vi "enqueue states.vi"(8 "error in (no error)":errorcluster, 10 "Wash Options":T1, 11 "Queue in":refnum<queue>) -> (0 "error out":errorcluster)   [LabVIEW 2015]
uses:
  Controls/Wash Options.ctl
  Controls/#status.ctl
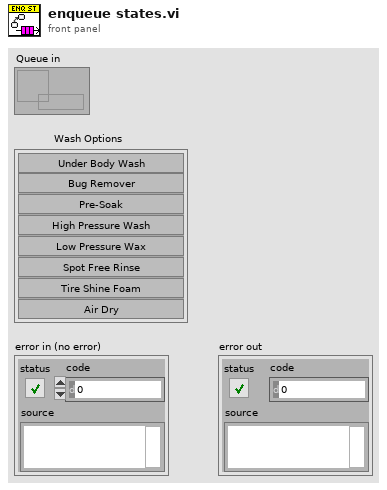
[diagram p1: front panel]
types:
  T1 = typedef "Wash Options.ctl" = cluster{"Underbody Wash":bool, "Bug Remover":bool, "Pre-Soak":bool, "High Pressure Wash":bool, "Low Pressure Wax":bool, "Spot Free Rinse":bool, "Tire Shine Foam":bool, "Air Dry":bool}
  T2 = typedef "#status.ctl" = enum16{"Error Under Range", "Skip", "Error", "Initialize", "End", "Air Dry", "Tire Shine Foam", "Spot Free Rinse", "Low Pressure Wax", "High Pressure Wash", "Pre-Soak", "Bug Remover", "Under Body Wash", "Start", "Idle", "Exit"}
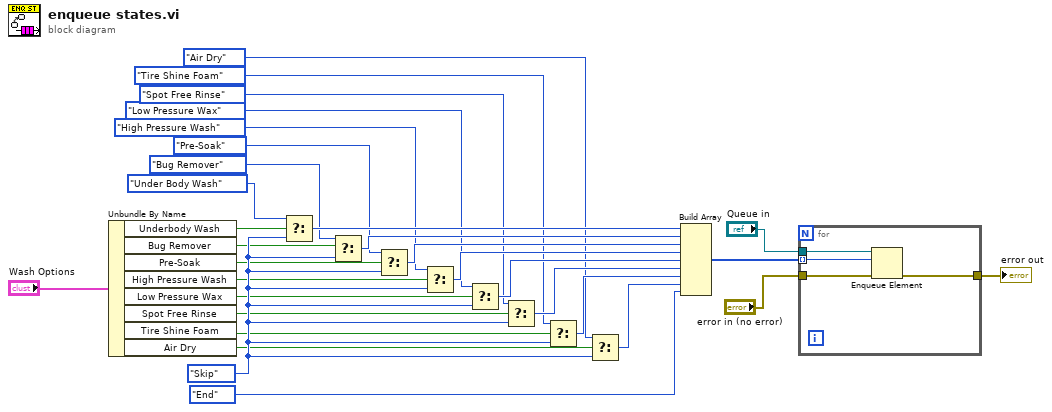
[diagram p0: block diagram]
diagram:
  w19 = #status."Skip" ("status")
  n1 = Unbundle By Name("Wash Options") -> ("Underbody Wash"=w3:bool, "Bug Remover"=w4:bool, "Pre-Soak"=w8:bool, "High Pressure Wash"=w12:bool, "Low Pressure Wax"=w13:bool, "Spot Free Rinse"=w14:bool, "Tire Shine Foam"=w15:bool, "Air Dry"=w16:bool)
  n2 = Select(t=#status."Under Body Wash" ("status"), s=w3, f=w19) -> (s? t:f=w20:T2)
  n3 = Select(t=#status."Bug Remover" ("status"), s=w4, f=w19) -> (s? t:f=w21:T2)
  n4 = Select(t=#status."Pre-Soak" ("status"), s=w8, f=w19) -> (s? t:f=w22:T2)
  n5 = Select(t=#status."High Pressure Wash" ("status"), s=w12, f=w19) -> (s? t:f=w23:T2)
  n6 = Select(t=#status."Low Pressure Wax" ("status"), s=w13, f=w19) -> (s? t:f=w24:T2)
  n7 = Select(t=#status."Spot Free Rinse" ("status"), s=w14, f=w19) -> (s? t:f=w25:T2)
  n8 = Select(t=#status."Tire Shine Foam" ("status"), s=w15, f=w19) -> (s? t:f=w26:T2)
  n9 = Select(t=#status."Air Dry" ("status"), s=w16, f=w19) -> (s? t:f=w27:T2)
  n10 = Build Array(w20, w21, w22, w23, w24, w25, w26, w27, #status."End" ("status")) -> (w28:T2[])
  n11 = for {
    tunnel: w28 -> [w35] mode=indexing
    tunnel: "error in (no error)" -> [w34]
    tunnel: [w33] -> w30
    tunnel: "Queue in" -> [w32]
    n12 = Enqueue Element(queue=w32, element=w35, error in (no error)=w34) -> (error out=w33:errorcluster)  [unwired: 1 in, 2 out]
  }
  "error out" <- w30
